vi "sample7(DXL).vi"() -> ()   [LabVIEW 2011]
panel:
  out "ModelInfo":T1
  out "rpm":dbl
  out "current":dbl
  out "angle":dbl
  out "success":bool
  in  "mode":u8(ring)=3 items=["OpCurrent"=0, "OpWheel"=1, "OpJoint"=3, "OpJointEx1"=4, "OpJointEx2"=5, "OpPWM"=16]
  out "ErrorCode":u16 format="%04x"
  in  "ID":u8=1 max=253
  in  "Baudrate":u32=57600 min=9600 max=12000000
  in  "COM":refnum<visa-resource-name> caption="COMポート"
  in  "STOP":bool
  in  "Value":dbl(knob) scale=720.0..-720.0
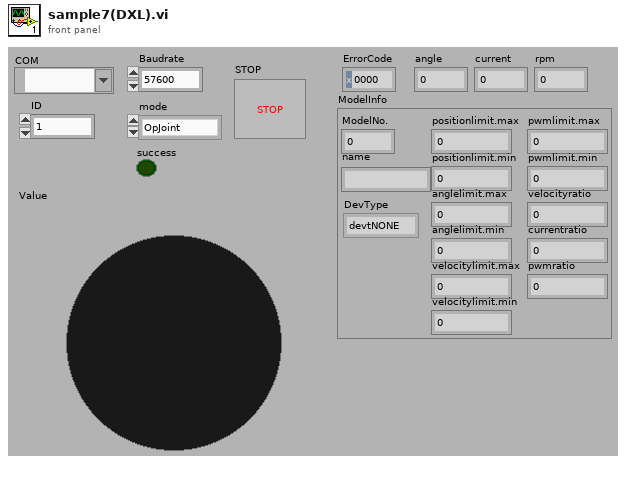
[diagram p1: front panel]
types:
  T1 = cluster{"ModelNo.":u16, "name":string, "DevType":enum32{"devtNONE", "devtDX", "devtAX", "devtRX", "devtEX", "devtMX", "devtXL320", "devtPRO", "devtX"}, "positionlimit.max":i32, "positionlimit.min":i32, "anglelimit.max":dbl, "anglelimit.min":dbl, "velocitylimit.max":i32, "velocitylimit.min":i32, "pwmlimit.max":i32, "pwmlimit.min":i32, "velocityratio":dbl, "currentratio":dbl, "pwmratio":dbl}
  T2 = enum32{"devtNONE", "devtDX", "devtAX", "devtRX", "devtEX", "devtMX", "devtXL320", "devtPRO", "devtX"}
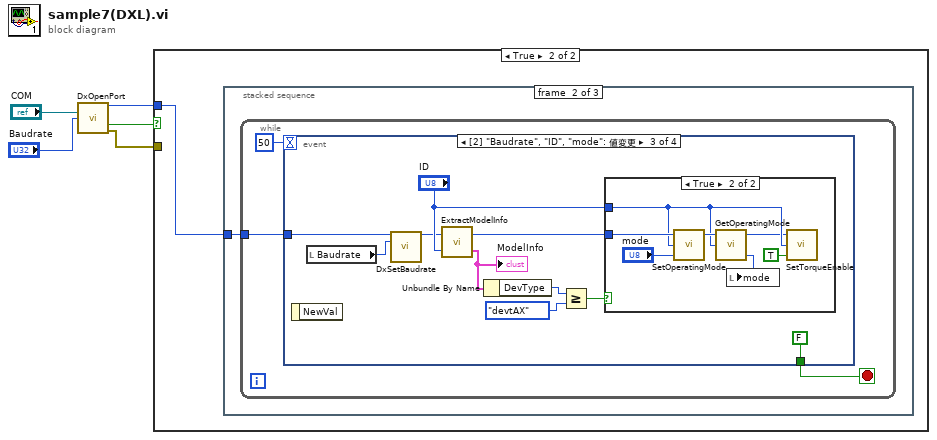
[diagram p0: block diagram]
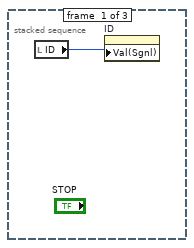
[diagram p3: hidden frame]
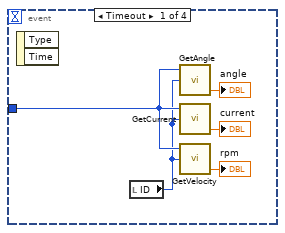
[diagram p4: hidden frame]
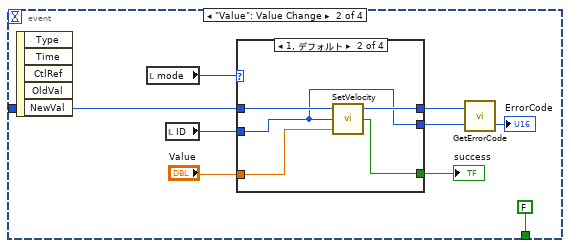
[diagram p5: hidden frame]
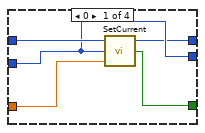
[diagram p6: hidden frame]
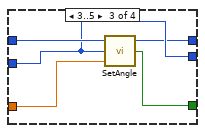
[diagram p7: hidden frame]
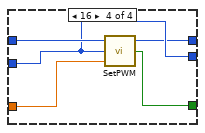
[diagram p8: hidden frame]
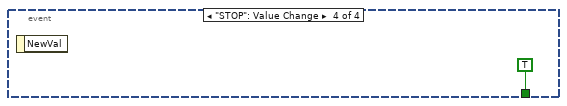
[diagram p10: hidden frame]
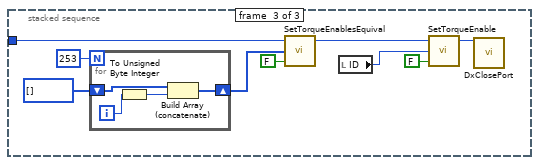
[diagram p11: hidden frame]
diagram:
  n1 = call "DxOpenPort.vi"("port"="COM", "baudrate"="Baudrate") -> ("dvid"=w3:u32, "成功"=w2:bool, "エラー出力"=w1:errorcluster)  [unwired: 11 in]
  n2 = case shown="TRUE" w2 {
    tunnel: w3 -> [_ w6]
    tunnel: w1 -> [_ _]
    frame False {
    }
    frame True {
      n3 = stacked-sequence {
        tunnel: w6 -> [_ w8 w65]
        frame #0 {
          n4 = local read "ID"() -> (w7:u8)
          n5 = property on="ID" class="DigNum （指定）"("Val(Sgnl)"=w7) -> ()  [unwired: 2 in, 2 out]
        }
        frame #1 {
          n6 = while {
            tunnel: w8 -> [w10]
            stop <- w9 stop-if-true
            n7 = event shown="[2] \"Baudrate\", \"ID\", \"mode\": 値変更" {
              selector: _ -> [_ _ _ _]
              dyn-events: _ -> [_ _ _ _]
              timeout: 50 -> [_ _ _ _]
              tunnel: w10 -> [w16 w23 w47 _]
              tunnel: [_ FALSE FALSE TRUE] -> w9
              event Timeout {
                n8 = event-data() -> ()  [unwired: 1 in, 2 out]
                n9 = local read "ID"() -> (w15:u8)
                n10 = call "GetAngle.vi"("Target ID"=w15, "dvid in"=w16) -> ("angle"=→"angle":dbl)  [unwired: 1 in, 2 out]
                n11 = call "GetCurrent.vi"("Target ID"=w15, "dvid in"=w16) -> ("current"=→"current":dbl)  [unwired: 1 in, 2 out]
                n12 = call "GetVelocity.vi"("Target ID"=w15, "dvid in"=w16) -> ("deg/s"=→"rpm":dbl)  [unwired: 1 in, 2 out]
              }
              event "Value": Value Change {
                n13 = event-data() -> ()  [unwired: 1 in, 5 out]
                n14 = local read "mode"() -> (w24:u8)
                n15 = local read "ID"() -> (w22:u8)
                n16 = case shown="1, デフォルト" w24 {
                  tunnel: w23 -> [w30 w35 w40 w45]
                  tunnel: w22 -> [w29 w33 w39 w44]
                  tunnel: [w28 w34 w38 w42] -> w20
                  tunnel: [w29 w33 w39 w44] -> w19
                  tunnel: "Value" -> [w27 w32 w37 w43]
                  tunnel: [w26 w31 w36 w41] -> w17
                  frame 0 {
                    n17 = call "SetCurrent.vi"("current"=w27, "Target ID"=w29, "dvid in"=w30) -> ("success"=w26:bool, "dvid out"=w28:u32)  [unwired: 1 in]
                  }
                  frame 1, Default {
                    n18 = call "SetVelocity.vi"("deg/s"=w32, "Target ID"=w33, "dvid in"=w35) -> ("success"=w31:bool, "dvid out"=w34:u32)  [unwired: 1 in]
                  }
                  frame 3..5 {
                    n19 = call "SetAngle.vi"("angle"=w37, "Target ID"=w39, "dvid in"=w40) -> ("success"=w36:bool, "dvid out"=w38:u32)  [unwired: 1 in]
                  }
                  frame 16 {
                    n20 = call "SetPWM.vi"("PWM"=w43, "Target ID"=w44, "dvid in"=w45) -> ("success"=w41:bool, "dvid out"=w42:u32)  [unwired: 1 in]
                  }
                }
                "success" <- w17
                n21 = call "GetErrorCode.vi"("Target ID"=w19, "dvid in"=w20) -> ("ErrorCode"=→"ErrorCode":u16)  [unwired: 1 out]
              }
              event "Baudrate", "ID", "mode": Value Change {
                n22 = event-data() -> ()  [unwired: 1 in, 1 out]
                n23 = local read "Baudrate"() -> (w48:u32)
                n24 = call "DxSetBaudrate.vi"("dvid in"=w47, "Baudrate"=w48) -> ("dvid out"=w46:u32)  [unwired: 11 in, 2 out]
                n25 = call "ExtractModelInfo.vi"("Target ID"="ID", "dvid in"=w46) -> ("ModelInfo"=w53:T1, "dvid out"=w55:u32)
                "ModelInfo" <- w53
                n26 = Unbundle By Name(w53) -> ("DevType"=w52:T2)
                n27 = Greater Or Equal?(x=w52, y=T2."devtAX" ("DevType")) -> (x >= y?=w50:bool)
                n28 = case shown="TRUE" w50 {
                  tunnel: w55 -> [_ w61]
                  tunnel: "ID" -> [_ w60]
                  frame False {
                  }
                  frame True {
                    n29 = call "SetOperatingMode.vi"("mode"="mode", "Target ID"=w60, "dvid in"=w61) -> ("dvid out"=w62:u32)  [unwired: 1 in, 1 out]
                    n30 = call "GetOperatingMode.vi"("Target ID"=w60, "dvid in"=w62) -> ("mode"=w56:u8, "dvid out"=w57:u32)  [unwired: 1 in, 1 out]
                    n31 = local write "mode"(w56) -> ()
                    n32 = call "SetTorqueEnable.vi"("torqueenable"=TRUE, "Target ID"=w60, "dvid in"=w57) -> ()  [unwired: 1 in, 2 out]
                  }
                }
              }
              event "STOP": Value Change {
                n33 = event-data() -> ()  [unwired: 1 in, 1 out]
              }
            }
          }
        }
        frame #2 {
          n34 = for {
            N: 253 -> [_]
            shift-right: [w75] -> w67
            shift-left: u8[] [] -> [w76]
            i -> [w74]
            n35 = To Unsigned Byte Integer(number=w74) -> (unsigned 8bit integer=w73:u8)
            n36 = Build Array (concatenate)(w76, w73) -> (w75:u8[])
          }
          n37 = call "SetTorqueEnablesEquival.vi"("torqueenable"=FALSE, "TargetIDs"=w67, "dvid in"=w65) -> ("dvid out"=w64:u32)  [unwired: 1 in, 1 out]
          n38 = local read "ID"() -> (w70:u8)
          n39 = call "SetTorqueEnable.vi"("torqueenable"=FALSE, "Target ID"=w70, "dvid in"=w64) -> ("dvid out"=w72:u32)  [unwired: 1 in, 1 out]
          n40 = call "DxClosePort.vi"("dvid"=w72) -> ()  [unwired: 13 in, 2 out]
        }
      }
    }
  }
